vi "Tlistener-1.vi"() -> ()   [LabVIEW 2015]
uses:
  <vilib>/Utility/error.llb/DialogType.ctl
  <vilib>/DAQmx/write.llb/DAQmx Write (Analog 1D DBL NChan 1Samp).vi
  <vilib>/DAQmx/create/channels.llb/DAQmx Create Channel (AO-Voltage-Basic).vi
  <vilib>/DAQmx/miscellaneous.llb/DAQmx Fill In Error Info.vi
panel:
  out "Warning container":enum32{"Warning", "No Warning"}(tab)
  in  "Local":bool=TRUE
  out "?":bool
  out "# Actions":i16
  in  "stop":bool
  in  "DataSocket Location":string="dstp://localhost/currentsources"
  in  "ADC channel":tag="Dev1/ao16:31"
  in  "Tuning state":dbl[](array[slide]) scale=0.0..10.0
  # "0\n1\n2\n3\n4\n5\n6\n7\n8\n9\n10\n11\n12\n13\n14\n15\n16\n17\n18\n19\n20\n21\n22\n23\n24\n25\n26\n27\n28\n29\n30\n31"
  # "WARNING: maximum voltage set to 10!!!\nGold Metals ONLY"
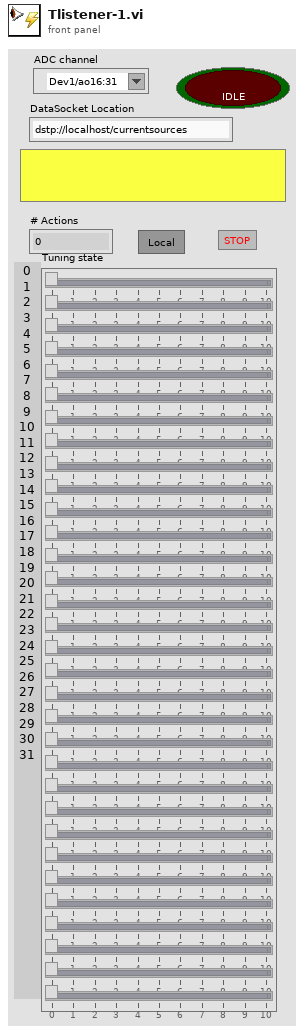
[diagram p1: front panel]
types:
  T1 = typedef "DialogType.ctl" = u16
  T2 = enum16{"Read", "Write", "ReadWrite", "BufferedRead", "BufferedReadWrite"}
  T3 = enum8{"Enabled", "Disabled", "Disabled and Grayed Out"}
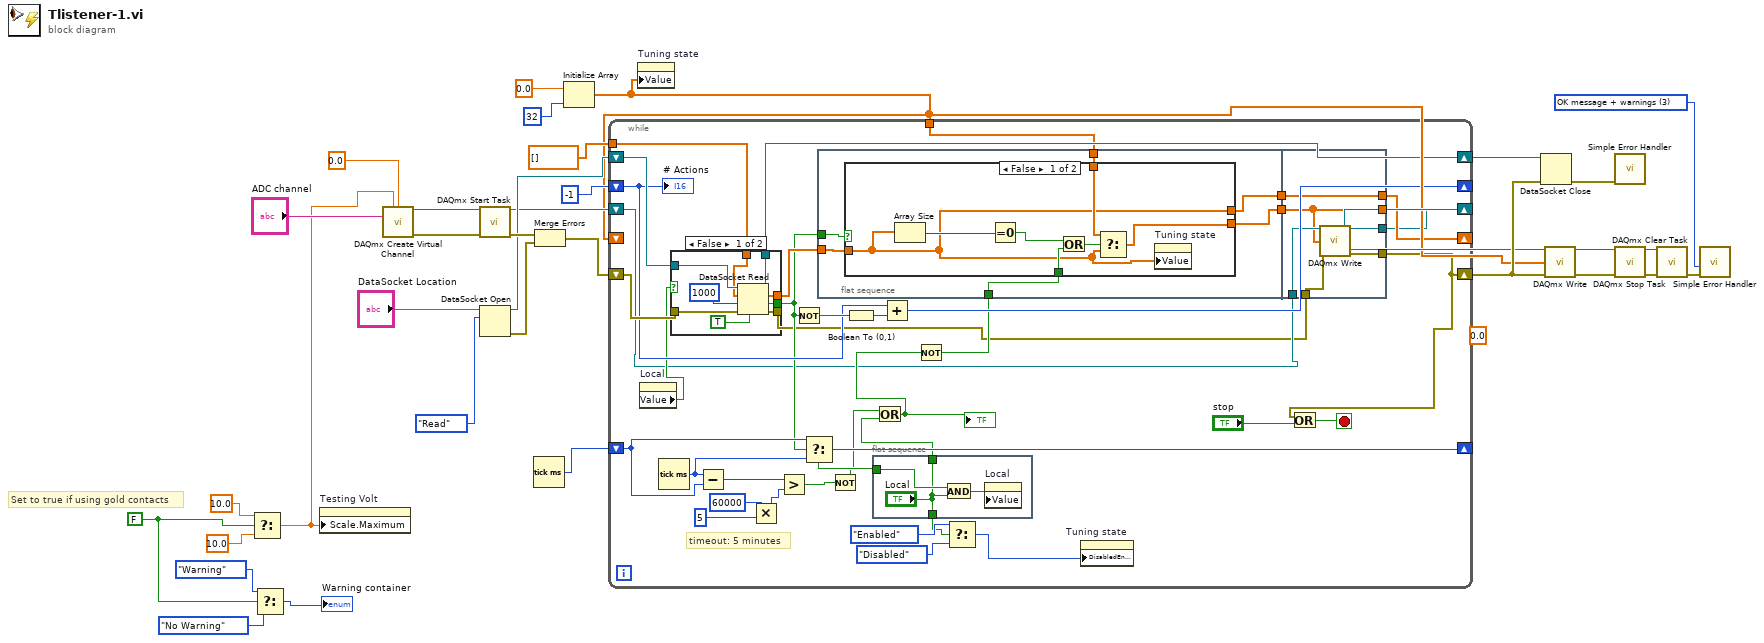
[diagram p0: block diagram]
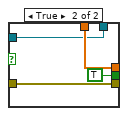
[diagram p2: hidden frame]
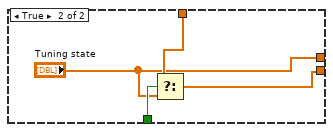
[diagram p3: hidden frame]
diagram:
  w3 = FALSE
  (unwired) 0.0 ("Waveform")
  w20 = T1 3 items=["no dialog", "OK message", "continue or stop message", "OK message + warnings", "continue/stop + warnings"] ("type of dialog (OK msg:1)")
  # "Set to true if using gold contacts"
  n1 = Select(t=10.0 ("maximum value"), s=w3, f=10.0) -> (s? t:f=w1:dbl)
  n2 = Select(t=enum32{"Warning", "No Warning"}."Warning" ("Warning container"), s=w3, f=enum32{"Warning", "No Warning"}."No Warning" ("Warning container")) -> (s? t:f=→"Warning container":enum32{"Warning", "No Warning"})
  n3 = property on="Testing Volt" class="Slide (strict)"("Scale.Maximum"=w1) -> ()  [unwired: 2 in, 2 out]
  n4 = call-poly <vilib>:"DAQmx Create Virtual Channel.vi"("maximum value"=w1, "minimum value"=0.0, "physical channels"="ADC channel") -> ("task out"=w33:refnum<k21>, "error out"=w32:errorcluster)  [unwired: 11 in]
  n5 = call <vilib>:"DAQmx Start Task.vi"("task/channels in"=w33, "error in"=w32) -> ("task out"=w23:refnum<k21>, "error out"=w27:errorcluster)  [unwired: 12 in]
  n6 = DataSocket Open(10:T2."Read" ("mode"), 11:"DataSocket Location") -> (0:w28:errorcluster, 3:w25:refnum<k13>)  [unwired: 2 in]
  n7 = Tick Count (ms)() -> (millisecond timer value=w11:u32)
  n8 = Merge Errors(w27, w28) -> (w26:errorcluster)
  n9 = Initialize Array(0.0 ("Waveform"), 32 ("dimension size")) -> (w2:dbl[])
  n10 = while {
    shift-right: [w39] -> w14
    shift-left: w26 -> [w68]
    tunnel: dbl[] [] -> [w67]
    shift-right: [w66] -> w15
    shift-left: w25 -> [w69]
    shift-right: [w38] -> w13
    shift-left: w23 -> [w41]
    shift-right: [w56] -> _
    shift-left: w2 -> [_]
    shift-right: [w61] -> _
    shift-left: i16 -1 -> [w62]
    shift-right: [w60] -> _
    shift-left: w11 -> [w58]
    tunnel: w2 -> [w44]
    stop <- w71 stop-if-true
    # "timeout: 5 minutes"
    n11 = property on="Local" class="Bool (strict)"() -> ("Value"=w45:bool)  [unwired: 2 in, 2 out]
    n12 = Tick Count (ms)() -> (millisecond timer value=w57:u32)
    n13 = case shown="False" w45 {
      tunnel: w69 -> [w79 w83]
      tunnel: w68 -> [w78 w82]
      tunnel: w67 -> [w77 w84]
      tunnel: [w76 w83] -> w66
      tunnel: [w75 w82] -> w40
      tunnel: [w74 w84] -> w65
      tunnel: [w72 TRUE ("timed out")] -> w51
      frame False {
        n14 = DataSocket Read(6:TRUE ("wait for updated value (T)"), 8:w78, 9:1000 ("ms timeout (10000)"), 10:w77, 11:w79) -> (0:w75:errorcluster, 1:w72:bool, 2:w74:dbl[], 3:w76:refnum<k13>)  [unwired: 3 out]
      }
      frame True {
      }
    }
    n15 = Subtract(x=w57, y=w58) -> (x-y=w59:u32)
    n16 = Multiply(x=u32 60000 ("y"), y=u32 5) -> (x*y=w36:u32)
    n17 = Greater?(x=w59, y=w36) -> (0:w48:bool)
    n18 = Not(x=w51) -> (.not. x?=w64:bool)
    n19 = Select(t=w58, s=w51, f=w57) -> (s? t:f=w60:u32)
    n20 = flat-sequence {
      tunnel: w65 -> [w89]
      tunnel: w51 -> [w90]
      tunnel: w46 -> [w87]
      tunnel: w44 -> [w86]
      tunnel: [w88] -> w43
      tunnel: [w85] -> w42
      tunnel: [w102] -> _
      tunnel: [w107] -> w56
      tunnel: w43 -> [w107]
      tunnel: w42 -> [w102]
      tunnel: w41 -> [w106]
      tunnel: w40 -> [w105]
      tunnel: [w104] -> w39
      tunnel: [w103] -> w38
      frame #0 {
        n21 = case shown="False" w90 {
          tunnel: w89 -> [w92 _]
          tunnel: [w92 "Tuning state"] -> w88
          tunnel: w87 -> [w95 w101]
          tunnel: w86 -> [w93 w100]
          tunnel: [w91 w98] -> w85
          frame False {
            n22 = Array Size(array=w92) -> (size(s)=w96:i32)
            n23 = Equal To 0?(x=w96) -> (x = 0?=w97:bool)
            n24 = Or(x=w97, y=w95) -> (x .or. y?=w94:bool)
            n25 = Select(t=w93, s=w94, f=w92) -> (s? t:f=w91:dbl[])
            n26 = property on="Tuning state" class="Arr (strict)"("Value"=w92) -> ()  [unwired: 2 in, 2 out]
          }
          frame True {
            n27 = Select(t=w100, s=w101, f="Tuning state") -> (s? t:f=w98:dbl[])
          }
        }
      }
      frame #1 {
        n28 = call-poly <vilib>:"DAQmx Write.vi"("task/channels in"=w106, "data"=w102, "error in"=w105) -> ("task out"=w103:refnum<k21>, "error out"=w104:errorcluster)  [unwired: 10 in, 1 out]
      }
    }
    n29 = Not(x=w48) -> (.not. x?=w50:bool)
    n30 = Boolean To (0,1)(Boolean=w64) -> (0, 1=w63:i16)
    n31 = flat-sequence {
      tunnel: ["Local"] -> w52
      tunnel: w51 -> [w109]
      tunnel: ["Local"] -> w49
      frame #0 {
        n32 = And(x=w109, y="Local") -> (x .and. y?=w110:bool)
        n33 = property on="Local" class="Bool (strict)"("Value"=w110) -> ()  [unwired: 2 in, 2 out]
      }
    }
    n34 = Or(x=w50, y=w49) -> (x .or. y?=w47:bool)
    "?" <- w47
    n35 = Add(x=w62, y=w63) -> (x+y=w61:i16)
    n36 = Not(x=w47) -> (.not. x?=w46:bool)
    n37 = Select(t=T3."Enabled" ("Disabled"), s=w52, f=T3."Disabled" ("Disabled")) -> (s? t:f=w55:T3)
    n38 = property on="Tuning state" class="Arr (strict)"("DisabledEnum"=w55) -> ()  [unwired: 2 in, 2 out]
    n39 = Or(x=w39, y="stop") -> (x .or. y?=w71:bool)
    "# Actions" <- w62
  }
  n40 = property on="Tuning state" class="Arr (strict)"("Value"=w2) -> ()  [unwired: 2 in, 2 out]
  n41 = DataSocket Close(8:w14, 11:w15) -> (0:w16:errorcluster)  [unwired: 1 in, 1 out]
  n42 = call-poly <vilib>:"DAQmx Write.vi"("task/channels in"=w13, "data"=w2, "error in"=w14) -> ("task out"=w21:refnum<k21>, "error out"=w22:errorcluster)  [unwired: 10 in, 1 out]
  n43 = call <vilib>:"Simple Error Handler.vi"("error in (no error)"=w16) -> ()  [unwired: 4 in, 5 out]
  n44 = call <vilib>:"DAQmx Stop Task.vi"("task/channels in"=w21, "error in"=w22) -> ("task out"=w18:refnum<k21>, "error out"=w19:errorcluster)  [unwired: 12 in]
  n45 = call <vilib>:"DAQmx Clear Task.vi"("task in"=w18, "error in"=w19) -> ("error out"=w17:errorcluster)  [unwired: 13 in]
  n46 = call <vilib>:"Simple Error Handler.vi"("type of dialog (OK msg:1)"=w20, "error in (no error)"=w17) -> ()  [unwired: 3 in, 5 out]
